vi "Servo host.vi"() -> ()   [LabVIEW 2009]
uses:
  <vilib>/rvi/interface/nirviOpenFPGA/nirviOpenFPGA.xnode
  FPGA Bitfiles/Servo.lvproj_FPGA Target_Servo.vi.lvbitx
  Servo.vi
  <vilib>/FPGAPlugInAG/cRIO-9104/nirviIntfOpen_cRIO-9104.vi
  <vilib>/rvi/interface/nirviMethod/nirviMethod.xnode
  <vilib>/rvi/interface/common/niFpgaNodeNameForErrorReporting.ctl
  <vilib>/rvi/errors/niLvFpgaWhatHappensToTopLevelVI.ctl
  <vilib>/Utility/error.llb/Error Cluster From Error Code.vi
  <vilib>/RVI Host/nirviSupport.llb/nirviErrorClusterFromErrorCode.vi
  <vilib>/LabVIEW Targets/FPGA/Rio/nirio_HostInterface/nirio_EnableInterrupts.vi
  <vilib>/rvi/errors/niLvFpgaReportInternalErrorWithAdditionalInfo.vi
  <vilib>/rvi/errors/niLvFpgaAdjustHostInterfaceError.vi
  <vilib>/rvi/interface/nirviReadWriteControl/nirviReadWriteControl.xnode
  <vilib>/rvi/interface/nirviCloseFPGA/nirviCloseFPGA.xnode
  <vilib>/FPGAPlugInAG/cRIO-9104/nirviIntfClose_cRIO-9104.vi
  <vilib>/userdefined/High Color/nirio_resource_hc.ctl
  NiRioSrv.dll
panel:
  in  "Select":enum16{"User defined", "Sine"}(ring)
  in  "Angle (deg)":dbl(slide) scale=-90.0..90.0
  in  "Stop":bool
  out "pulse width (us)":i32
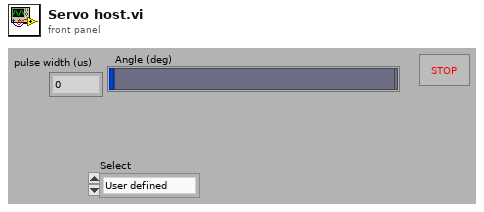
[diagram p1: front panel]
types:
  T1 = typedef "niFpgaNodeNameForErrorReporting.ctl" = enum16{"Open FPGA VI Reference", "Read/Write Control", "Invoke Method: Abort", "Invoke Method: Acknowledge IRQ", "Invoke Method: Download", "Invoke Method: FIFO.Configure", "Invoke Method: FIFO.Read", "Invoke Method: FIFO.Start", "Invoke Method: FIFO.Stop", "Invoke Method: FIFO.Write", "Invoke Method: Reset", "Invoke Method: Run", "Invoke Method: Wait on IRQ", "Close FPGA VI Reference"}
  T2 = typedef "niLvFpgaWhatHappensToTopLevelVI.ctl" = enum16{"top level VI scripted behind XNode", "top level VI inlined behind XNode"}
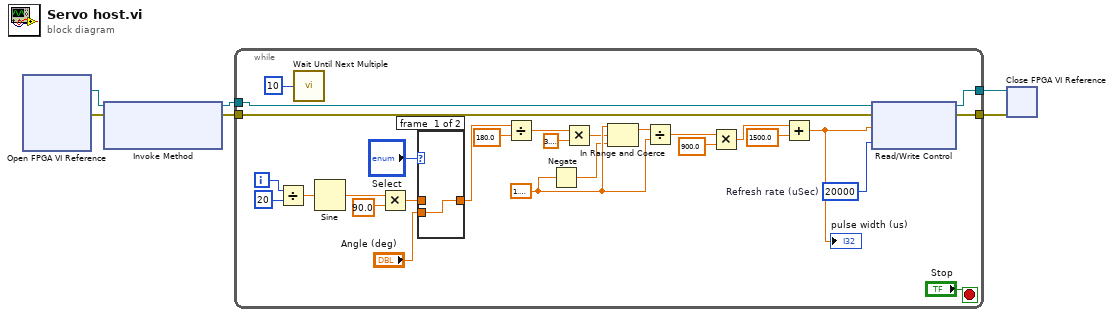
[diagram p0: block diagram]
diagram:
  n1 = xnode "Open FPGA VI Reference"() -> ("FPGA VI Reference Out"=w6:refnum<k20>, "error out"=w5:errorcluster)  [unwired: 2 in]
  n2 = xnode "Invoke Method"("FPGA VI Reference In"=w6, "error in"=w5) -> ("FPGA VI Reference Out"=w4:refnum<k20>, "error out"=w3:errorcluster)  [unwired: 1 out]
  n3 = while {
    tunnel: w4 -> [w34]
    tunnel: w3 -> [w33]
    tunnel: [w23] -> w2
    tunnel: [w22] -> w1
    i -> [w13]
    stop <- "Stop" stop-if-true
    w21 = u32 20000  # Refresh rate (uSec)
    w28 = 1.5707963267948966
    n4 = Divide(x=w13, y=20) -> (x/y=w12:dbl)
    n5 = call "Wait Until Next Multiple"("Count(mSec)"=u32 10) -> ()  [unwired: 1 out]
    n6 = Sine(x=w12) -> (sin(x)=w15:dbl)
    n7 = Multiply(x=w15, y=90.0) -> (x*y=w10:dbl)
    n8 = case shown="\"User defined\", Default" "Select" {
      tunnel: w10 -> [_ w36]
      tunnel: "Angle (deg)" -> [w35 _]
      tunnel: [w35 w36] -> w8
      frame #0 {
      }
      frame #1 {
      }
    }
    n9 = Divide(x=w8, y=180.0) -> (x/y=w19:dbl)
    n10 = Negate(x=w28) -> (-x=w26:dbl)
    n11 = Multiply(x=w19, y=3.141592653589793) -> (x*y=w18:dbl)
    n12 = In Range and Coerce(upper limit=w28, x=w18, lower limit=w26) -> (coerced(x)=w27:dbl)  [unwired: 1 out]
    n13 = Divide(x=w27, y=w28) -> (x/y=w29:dbl)
    n14 = Multiply(x=w29, y=900.0) -> (x*y=w31:dbl)
    n15 = Add(x=w31, y=1500.0) -> (x+y=w25:dbl)
    "pulse width (us)" <- w25
    n16 = xnode "Read/Write Control"("FPGA VI Reference In"=w34, "error in"=w33, "servo 6"=w25, "Count(uSec)"=w21) -> ("FPGA VI Reference Out"=w23:refnum<k20>, "error out"=w22:errorcluster)
  }
  n17 = xnode "Close FPGA VI Reference"("FPGA VI Reference In"=w2, "error in"=w1) -> ()  [unwired: 1 out]
